vi "Write Key.vi"(8 "error in (no error)":errorcluster, 11 "[MV] Key Certify in":refnum<class "[MV] Key Certify.lvclass">) -> (0 "error out":errorcluster, 3 "[MV] Key Certify out":refnum<class "[MV] Key Certify.lvclass">)   [LabVIEW 2023, in "[MV] Key Certify.lvlib" / "[MV] Key Certify.lvclass"]
uses:
  [MV] Key Certify.lvclass
  [MV] Key Certify.lvclass/[MV] Key Certify.ctl
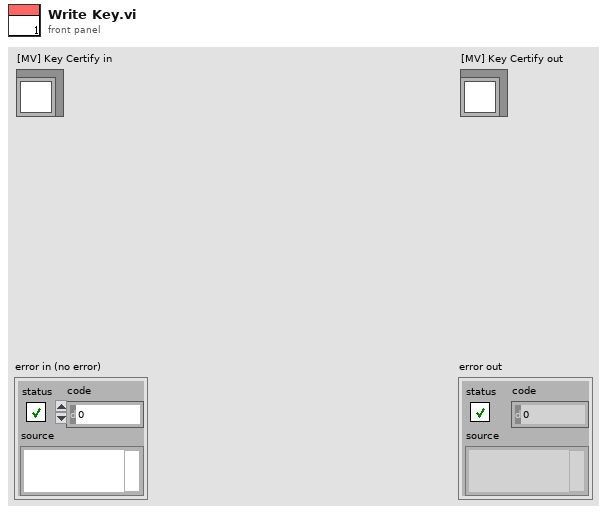
[diagram p1: front panel]
types:
  T1 = enum16{"open", "replace", "create", "open or create", "replace or create", "replace or create with confirmation"}
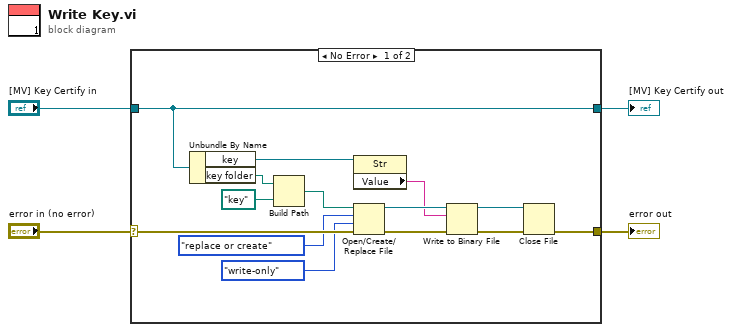
[diagram p0: block diagram]
diagram:
  n1 = case shown="No Error" "error in (no error)" {
    selector: "error in (no error)" -> [w17 w20]
    tunnel: [w7 w20] -> w3
    tunnel: [w18 w19] -> w1
    tunnel: "[MV] Key Certify in" -> [w18 w19]
    frame No Error {
      n2 = Unbundle By Name(w18) -> ("key"=w6:refnum<vi>, "key folder"=w16:path)
      n3 = Build Path(base path=w16, name or relative path=path "key") -> (appended path=w14:path)
      n4 = property class="Str"(reference=w6) -> ("Value"=w5:string)  [unwired: 1 in, 2 out]
      n5 = Open/Create/Replace File(file path (use dialog)=w14, error in=w17, operation (0:open)=T1."replace or create", access (0:read/write)=enum16{"read/write", "read-only", "write-only"}."write-only") -> (refnum out=w9:refnum<file>, error out=w11:errorcluster)  [unwired: 2 in, 1 out]
      n6 = Write to Binary File(file (use dialog)=w9, data=w5, error in=w11) -> (refnum out=w8:refnum<file>, error out=w10:errorcluster)  [unwired: 3 in, 1 out]
      n7 = Close File(refnum=w8, error in=w10) -> (error out=w7:errorcluster)  [unwired: 1 out]
    }
    frame Error {
    }
  }
  "error out" <- w3
  "[MV] Key Certify out" <- w1
